vi "Untitled 1.vi"(6 "KeyNumber":i32=52, 7 "WhiteKeySize":cluster{"Width":i32, "Hieght":i32}={"Width"=21, "Hieght"=147}, 8 "error in (no error)":errorcluster, 10 "音名Array":string[](array[string]), 11 "Image In":T1) -> (0 "error out":errorcluster, 3 "Image Out":T1)   [LabVIEW 2015]
uses:
  <vilib>/vision/Image Controls.llb/IMAQ Image.ctl
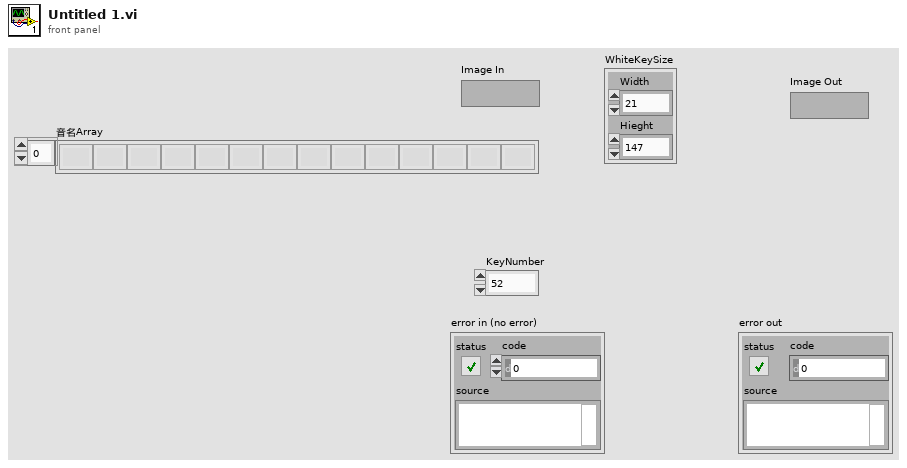
[diagram p1: front panel]
types:
  T1 = typedef "IMAQ Image.ctl" = refnum<image>
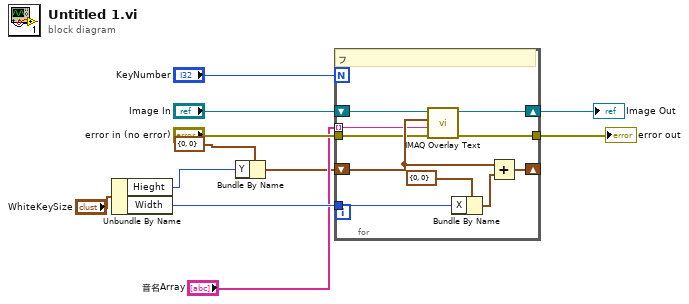
[diagram p0: block diagram]
diagram:
  n1 = Unbundle By Name("WhiteKeySize") -> ("Hieght"=w1:i32, "Width"=w6:i32)
  n2 = Bundle By Name(cluster=cluster{"X":i32, "Y":i32} {"X"=0, "Y"=0} ("Top Left Point"), "Y"=w1) -> (w2:cluster{"X":i32, "Y":i32})
  n3 = for {
    N: "KeyNumber" -> [_]
    shift-right: [w16] -> w8
    shift-left: "Image In" -> [w17]
    shift-right: [w21] -> _
    shift-left: w2 -> [w15]
    tunnel: w6 -> [w18]
    tunnel: "error in (no error)" -> [w13]
    tunnel: [w12] -> w9
    tunnel: "音名Array" -> [w14] mode=indexing
    # "フ"
    n4 = call "IMAQ Overlay Text"("error in (no error)"=w13, "String"=w14, "Origin"=w15, "Image"=w17) -> ("error out"=w12:errorcluster, "Image Out"=w16:T1)  [unwired: 6 in]
    n5 = Bundle By Name(cluster=cluster{"X":i32, "Y":i32} {"X"=0, "Y"=0} ("y"), "X"=w18) -> (w19:cluster{"X":i32, "Y":i32})
    n6 = Add(x=w15, y=w19) -> (x+y=w21:cluster{"X":i32, "Y":i32})
  }
  "Image Out" <- w8
  "error out" <- w9
